vi "Configure Chan Input.vi"(6 "Gate Mode (0:Disabled)":T1(ring), 7 "Channel (1:Chan A)":i32(ring)=1 items=["Channel A"=1, "Channel B"=2, "Channel C"=3, "Channel D"=4, "Channel E"=5, "Channel F"=6, "Channel G"=7, "Channel H"=8], 8 "error in (no error)":errorcluster, 9 "Gate Logic (0:Disabled)":enum16{"Disabled", "Low", "High"}(ring), 10 "Sync Source (0:To)":i32(ring) items=["System (To)", "Channel A", "Channel B", "Channel C", "Channel D", "Channel E", "Channel F", "Channel G", "Channel H"], 11 "VISA resource name":refnum<visa-resource-name>) -> (0 "error out":errorcluster, 3 "VISA resource name out":refnum<visa-resource-name>)   [LabVIEW 2019, in "Quantum Composers 9000 Series.lvlib"]
doc: "This VI is used to configure the gate mode for a channel."
uses:
  Quantum Composers 9000 Series.lvlib
panel:
  out "Read Buffer":string
  # "The \"Gate Mode\" input is currently only utilized by 9520/9530 instruments.  When controlling a 9520/9530, the \"Gate Logic\" disabled setting is ignored."
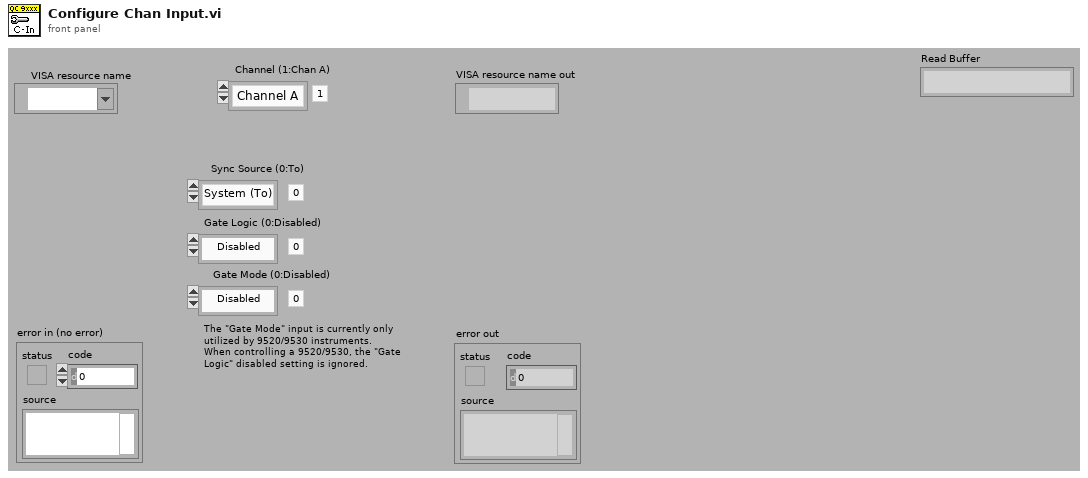
[diagram p1: front panel]
types:
  T1 = enum16{"Disabled", "Pulse Inhibit", "Output Inhibit"}
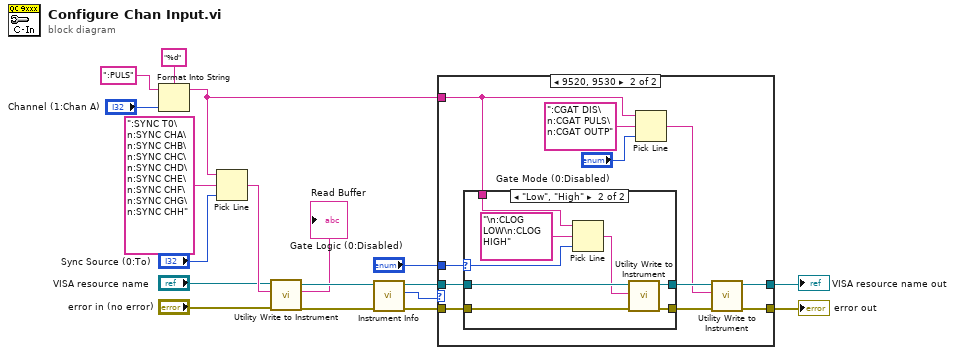
[diagram p0: block diagram]
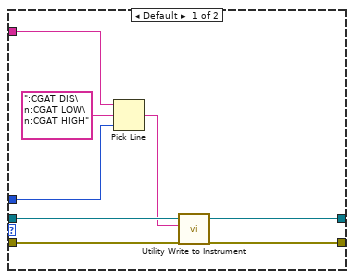
[diagram p2: hidden frame]
diagram:
  n1 = Format Into String(format string="%d", initial string=":PULS", "Channel (1:Chan A)") -> (resulting string=w6:string)  [unwired: 1 in, 1 out]
  n2 = Pick Line(string ("")=w6, multi-line string=":SYNC T0\n:SYNC CHA\n:SYNC CHB\n:SYNC CHC\n:SYNC CHD\n:SYNC CHE\n:SYNC CHF\n:SYNC CHG\n:SYNC CHH", line index="Sync Source (0:To)") -> (output string=w16:string)
  n3 = call "Utility Write to Instrument.vi"("error in (no error)"="error in (no error)", "Write Buffer"=w16, "VISA resource name"="VISA resource name") -> ("error out"=w12:errorcluster, "Read Buffer"=→"Read Buffer":string, "VISA resource name out"=w11:refnum<visa-resource-name>)  [unwired: 6 in]
  n4 = call "Instrument Info.vi"("error in (no error)"=w12, "VISA resource name"=w11) -> ("error out"=w4:errorcluster, "Instr Model"=w2:u32, "VISA resource name out"=w5:refnum<visa-resource-name>)  [unwired: 6 in, 1 out]
  n5 = case shown="9520, 9530" w2 {
    tunnel: [w26 w35] -> w10
    tunnel: [w24 w34] -> w9
    tunnel: w6 -> [w21 w28]
    tunnel: w5 -> [w23 w36]
    tunnel: w4 -> [w25 w37]
    tunnel: "Gate Logic (0:Disabled)" -> [w19 w29]
    frame Default {
      n6 = Pick Line(string ("")=w21, multi-line string=":CGAT DIS\n:CGAT LOW\n:CGAT HIGH", line index=w19) -> (output string=w20:string)
      n7 = call "Utility Write to Instrument.vi"("error in (no error)"=w25, "Write Buffer"=w20, "VISA resource name"=w23) -> ("error out"=w26:errorcluster, "VISA resource name out"=w24:refnum<visa-resource-name>)  [unwired: 6 in, 1 out]
    }
    frame 9520, 9530 {
      n8 = case shown="\"Low\", \"High\"" w29 {
        selector: w29 -> [_ w41]
        tunnel: [w38 w47] -> w32
        tunnel: w37 -> [w38 w44]
        tunnel: [w39 w46] -> w33
        tunnel: w36 -> [w39 w45]
        tunnel: w28 -> [_ w42]
        frame "Disabled" {
        }
        frame "Low", "High" {
          n9 = Pick Line(string ("")=w42, multi-line string="\n:CLOG LOW\n:CLOG HIGH", line index=w41) -> (output string=w40:string)
          n10 = call "Utility Write to Instrument.vi"("error in (no error)"=w44, "Write Buffer"=w40, "VISA resource name"=w45) -> ("error out"=w47:errorcluster, "VISA resource name out"=w46:refnum<visa-resource-name>)  [unwired: 6 in, 1 out]
        }
      }
      n11 = Pick Line(string ("")=w28, multi-line string=":CGAT DIS\n:CGAT PULS\n:CGAT OUTP", line index="Gate Mode (0:Disabled)") -> (output string=w27:string)
      n12 = call "Utility Write to Instrument.vi"("error in (no error)"=w32, "Write Buffer"=w27, "VISA resource name"=w33) -> ("error out"=w35:errorcluster, "VISA resource name out"=w34:refnum<visa-resource-name>)  [unwired: 6 in, 1 out]
    }
  }
  "error out" <- w10
  "VISA resource name out" <- w9
